vi "Task Loop.vi"(8 "error in (no error)":errorcluster, 11 "DebugGUI in":refnum<class "DebugGUI.lvclass">) -> (0 "error out":errorcluster)   [LabVIEW 2020, in "Volatus.lvlib" / "DebugGUI.lvclass"]
uses:
  DebugGUI.lvclass
  C:/dev/lv20CE/relink/lv-volatus/Volatus/Task/Task.lvclass
  VolatusAPI/VolatusAPI.lvclass
  C:/dev/lv20CE/relink/lv-volatus/Volatus/API/API.lvclass
  DebugGUI.lvclass/DebugGUI.ctl
  Task/Task.lvclass/Task.ctl
  VolatusAPI/VolatusAPI.lvclass/VolatusAPI.ctl
  Identity/Key.vi
  <vilib>/Utility/error.llb/Error Cluster From Error Code.vi
  API/API.lvclass
  Identity/Identity.lvclass
  Task/Task.lvclass
panel:
  out "Tree":string(tree)
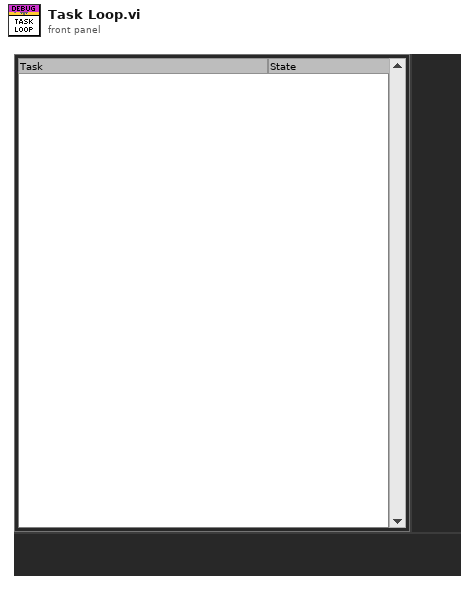
[diagram p1: front panel]
types:
  T1 = typedef "Volatus.lvlib/Task Run Info.ctl" = cluster{"Hierarchy":T2, "State":T3}
  T2 = typedef "Volatus.lvlib/Task Hierarchy.ctl" = string[]
  T3 = typedef "Volatus.lvlib/Task State.ctl" = enum16{"Unknown", "Idle", "Initializing", "Starting", "Running", "Stopping", "Stopped", "Error - Init", "Error - Start", "Error - Run", "Error - Stop"}
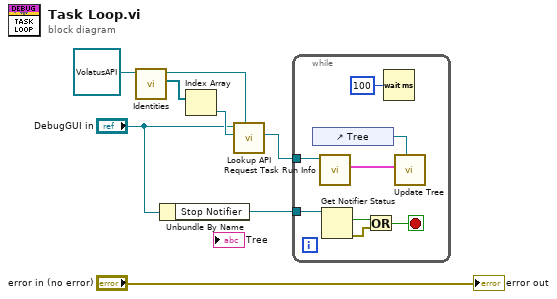
[diagram p0: block diagram]
diagram:
  n1 = call-dynamic "Identities.vi"("VolatusAPI in"=refnum<class "VolatusAPI.lvclass"> refnum ("Volatus:VolatusAPI")) -> ("Identities"=w5:refnum<class "Identity.lvclass">[], "VolatusAPI out"=w4:refnum<class "VolatusAPI.lvclass">)  [unwired: 8 in, 1 out]
  n2 = Unbundle By Name("DebugGUI in") -> ("Stop Notifier"=w1:refnum<notifier>)
  n3 = Index Array(array=w5) -> (element=w6:refnum<class "Identity.lvclass">)  [unwired: 1 in]
  n4 = call "Lookup API.vi"("API Type"=w4, "Identity"=w6, "Task in"="DebugGUI in") -> ("API"=w3:refnum<class "VolatusAPI.lvclass">)  [unwired: 6 in, 2 out]
  n5 = while {
    tunnel: w3 -> [w16]
    tunnel: w1 -> [w12]
    stop <- w9 stop-if-true
    n6 = control-ref of="Tree"() -> (w13:refnum<vi>)
    n7 = call "Request Task Run Info.vi"("VolatusAPI in"=w16) -> ("Task Run Info"=w14:T1[])  [unwired: 8 in, 2 out]
    n8 = Get Notifier Status(notifier=w12) -> (current notification=w10:bool, error out=w11:errorcluster)  [unwired: 1 in, 3 out]
    n9 = Or(x=w10, y=w11) -> (x .or. y?=w9:bool)
    n10 = Wait (ms)(milliseconds to wait=u32 100) -> ()  [unwired: 1 out]
    n11 = call "Update Tree.vi"("Tree"=w13, "Task Run Info"=w14) -> ()  [unwired: 9 in, 1 out]
  }
  "error out" <- "error in (no error)"
